vi "Globals.vi"() -> ()   [LabVIEW 2011]
panel:
  in  "MasterDIR":path
  out "DEC Tmp":dbl format="%<%H:%M:%S>t"
  out "RA Tmp":dbl format="%<%H:%M:%S%1u>t"
  in  "DEC_track":dbl format="%.3g"
  out "AD_track":dbl format="%.3g"
  out "Arrêt par offset":bool
  out "is running?":bool
  out "BonOMM VI Refnum":refnum<vi>
  out "CameraTuning VI Refnum":refnum<vi>
  out "Guiding starded":bool
  out "Y.agg":sgl
  out "X.agg":sgl
  out "EXIT":bool
  out "Image_miroir":i32[][](graph)
  out "StartGuide":bool
  out "Aborted":bool
  out "GuiderUpdate":bool
  in  "ScopeSim._Telescope":refnum<k7>
  in  "MaxIm.ICCDCamera":refnum<k7>
  out "GuidingStar":i32[][](graph)
  out "GuiderYError":sgl format="%.2f"
  out "GuiderXError":sgl format="%.2f"
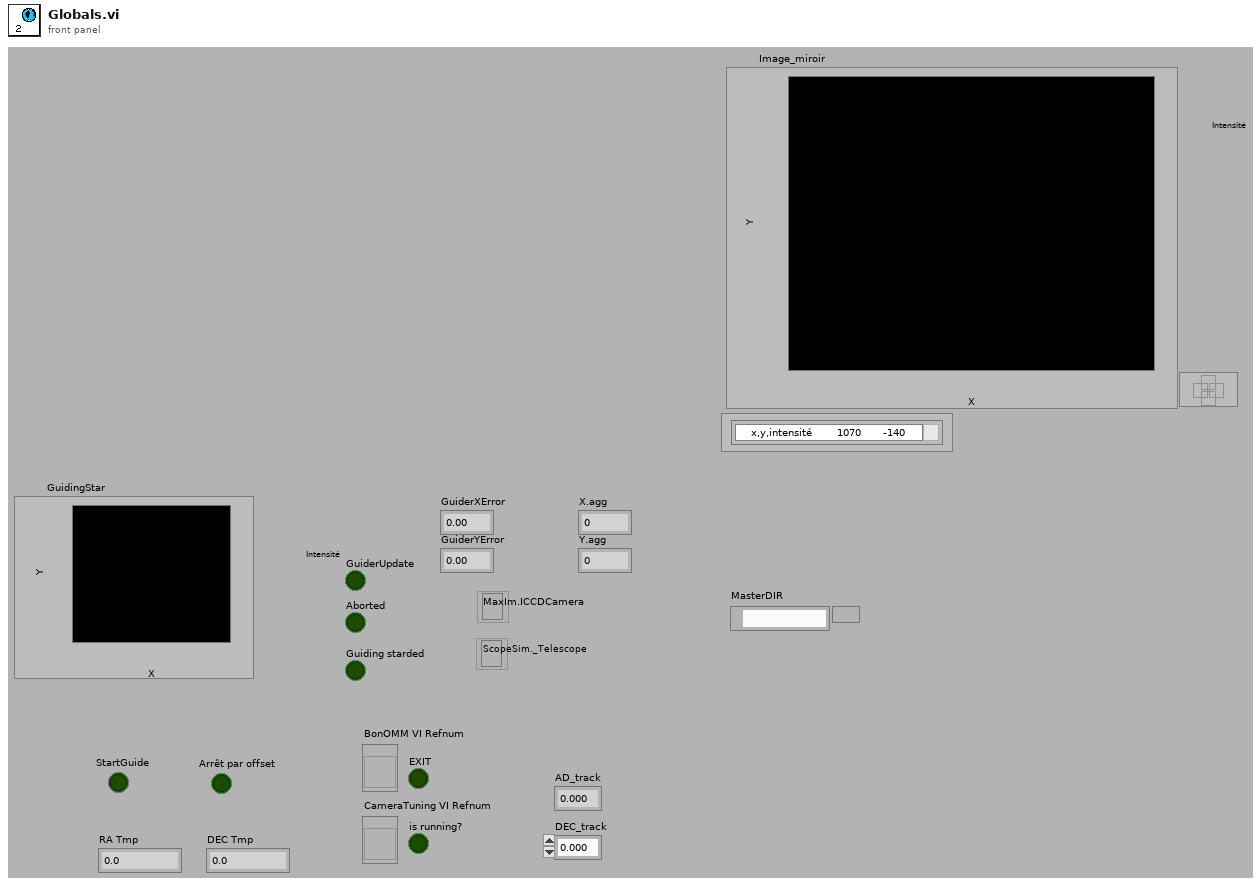
[diagram p1: front panel]
diagram:
